vi "Decimator Function.vi"(9 "Decimation #":i32, 10 "Input Y values New":dbl[](array[numeric]), 11 "Input Y values Old":dbl[](array[numeric])) -> (3 "Output Y Values":dbl[](array[numeric]))   [LabVIEW 2014]
panel:
  # "Decimator Function"
  # "Inputs"
  # "Outputs"
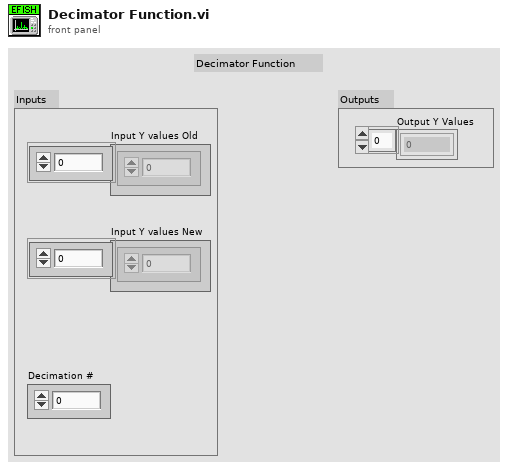
[diagram p1: front panel]
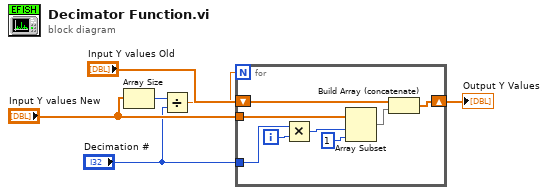
[diagram p0: block diagram]
diagram:
  n1 = Array Size(array="Input Y values New") -> (size(s)=w5:i32)
  n2 = Divide(x=w5, y="Decimation #") -> (x/y=w4:dbl)
  n3 = for {
    N: w4 -> [_]
    shift-right: [w7] -> w1
    shift-left: "Input Y values Old" -> [w8]
    tunnel: "Input Y values New" -> [w14]
    tunnel: "Decimation #" -> [w12]
    i -> [w13]
    n4 = Multiply(x=w12, y=w13) -> (x*y=w11:i32)
    n5 = Array Subset(array=w14, index=w11, length=1) -> (w9:dbl[])
    n6 = Build Array (concatenate)(w8, w9) -> (w7:dbl[])
  }
  "Output Y Values" <- w1
